vi "Apply Selected Labels to Control.vi"(8 "error in (no error)":errorcluster, 10 "Alternate Text Select (0)":i32, 11 "Enum in":refnum<class "Enum.lvclass">) -> (0 "error out":errorcluster, 3 "Enum out":refnum<class "Enum.lvclass">)   [LabVIEW 2017, in "Localization.lvlib" / "Enum.lvclass"]
doc: "Use the information in the class to apply the selected alternate text from the Additional Labels to the control.\n\nChoose Movement Consulting, LLC"
uses:
  Enum.lvclass
  C:/Apps/CMC/OpenSource/Localization/Control Info/Control Info.lvclass
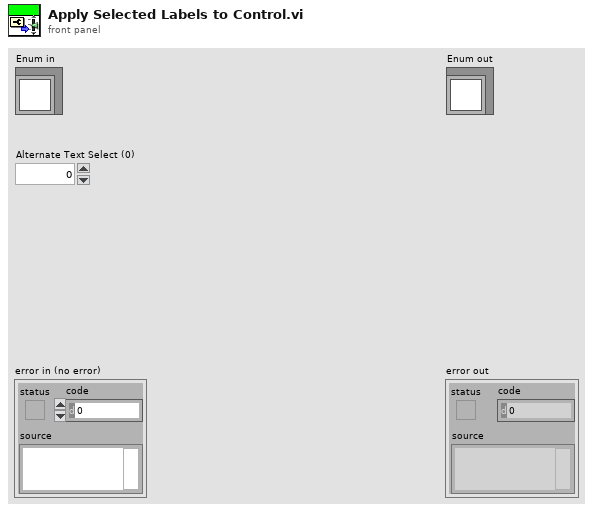
[diagram p1: front panel]
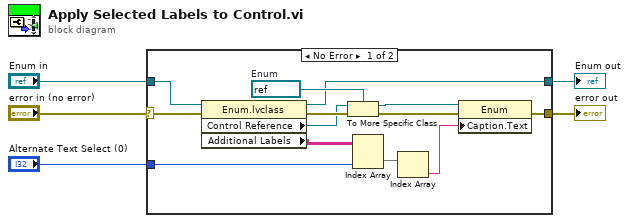
[diagram p0: block diagram]
diagram:
  n1 = case shown="No Error" "error in (no error)" {
    selector: "error in (no error)" -> [w13 w20]
    tunnel: "Enum in" -> [w12 w19]
    tunnel: [w7 w20] -> w4
    tunnel: [w6 w19] -> w1
    tunnel: "Alternate Text Select (0)" -> [w10 _]
    frame No Error {
      w18 = refnum<vi> refnum  # Enum
      n2 = property class="Enum.lvclass"(reference=w12, error in=w13) -> (reference out=w6:refnum<class "Enum.lvclass">, error out=w15:errorcluster, "Control Reference"=w14:refnum<vi>, "Additional Labels"=w11:string[][])
      n3 = To More Specific Class(target class=w18, reference=w14, error in=w15) -> (specific class reference=w17:refnum<vi>, error out=w16:errorcluster)
      n4 = Index Array(array=w11, index (col)=w10) -> (element=w8:string[])  [unwired: 1 in]
      n5 = Index Array(array=w8) -> (element=w9:string)  [unwired: 1 in]
      n6 = property class="Enum"(reference=w17, error in=w16, "Caption.Text"=w9) -> (error out=w7:errorcluster)  [unwired: 1 out]
    }
    frame Error {
    }
  }
  "error out" <- w4
  "Enum out" <- w1
